vi "Nov_30.vi"() -> ()   [LabVIEW 2020]
uses:
  <vilib>/Utility/error.llb/DialogType.ctl
  <vilib>/Analysis/3filter.llb/Filter Passband Type.ctl
  <vilib>/DAQmx/read.llb/DAQmx Read (Analog 1D DBL NChan 1Samp).vi
  <vilib>/DAQmx/create/channels.llb/DAQmx Create Channel (AI-Voltage-Basic).vi
  <vilib>/DAQmx/configure/timing.llb/DAQmx Timing (Sample Clock).vi
  <vilib>/DAQmx/miscellaneous.llb/DAQmx Fill In Error Info.vi
  <vilib>/Analysis/3filter.llb/Butterworth Filter (DBL).vi
  <vilib>/Utility/file.llb/Write Delimited Spreadsheet (string).vi
  <vilib>/Utility/file.llb/Write Delimited Spreadsheet (DBL).vi
  <vilib>/Analysis/NI_AALBase.lvlib
panel:
  in  "Motor Enable":bool
  out "Swing (Consumer Loop)":bool
  in  "Motor Trottle":dbl(slide) scale=0.0..5.0
  in  "Master Stop":bool
  out "Consumer Loop Speed":u32
  out "Producer Loop Speed":u32
  out "Swing":bool
  out "Force Plate":dynamicdata(graph)
  out "Accelerometers":dynamicdata(graph)
  out "Enlapsed Time (sec)":dbl
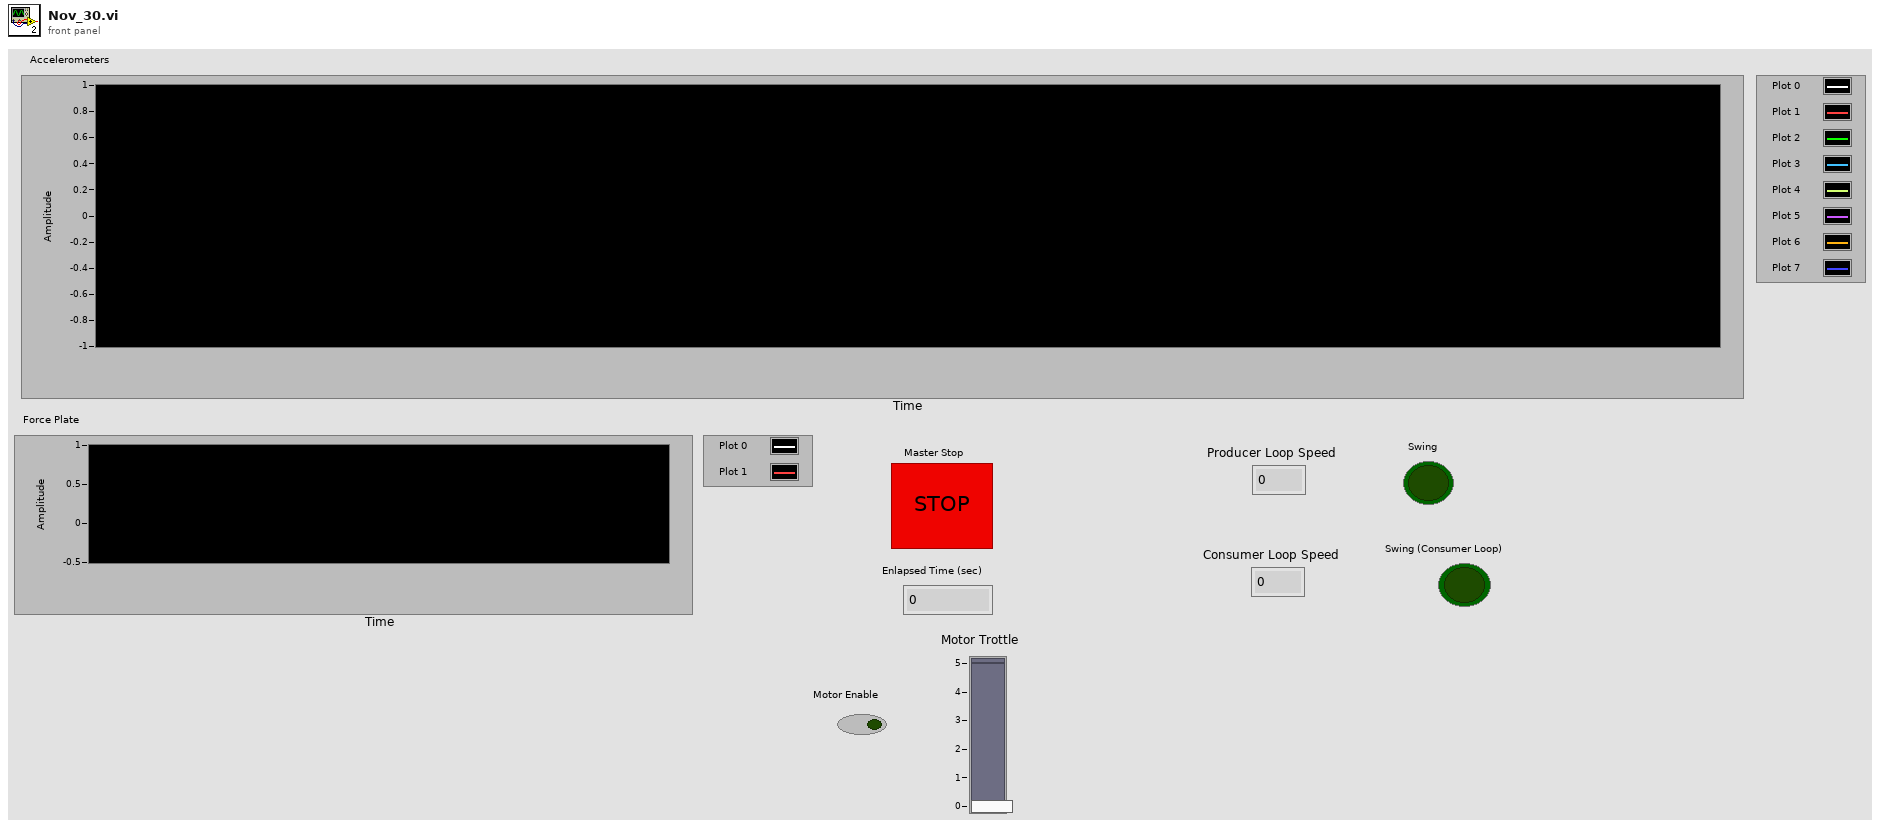
[diagram p1: front panel]
types:
  T1 = typedef "DialogType.ctl" = u16
  T2 = typedef "NI_AALBase.lvlib/Filter Passband Type.ctl" = enum32{"Lowpass", "Highpass", "Bandpass", "Bandstop"}
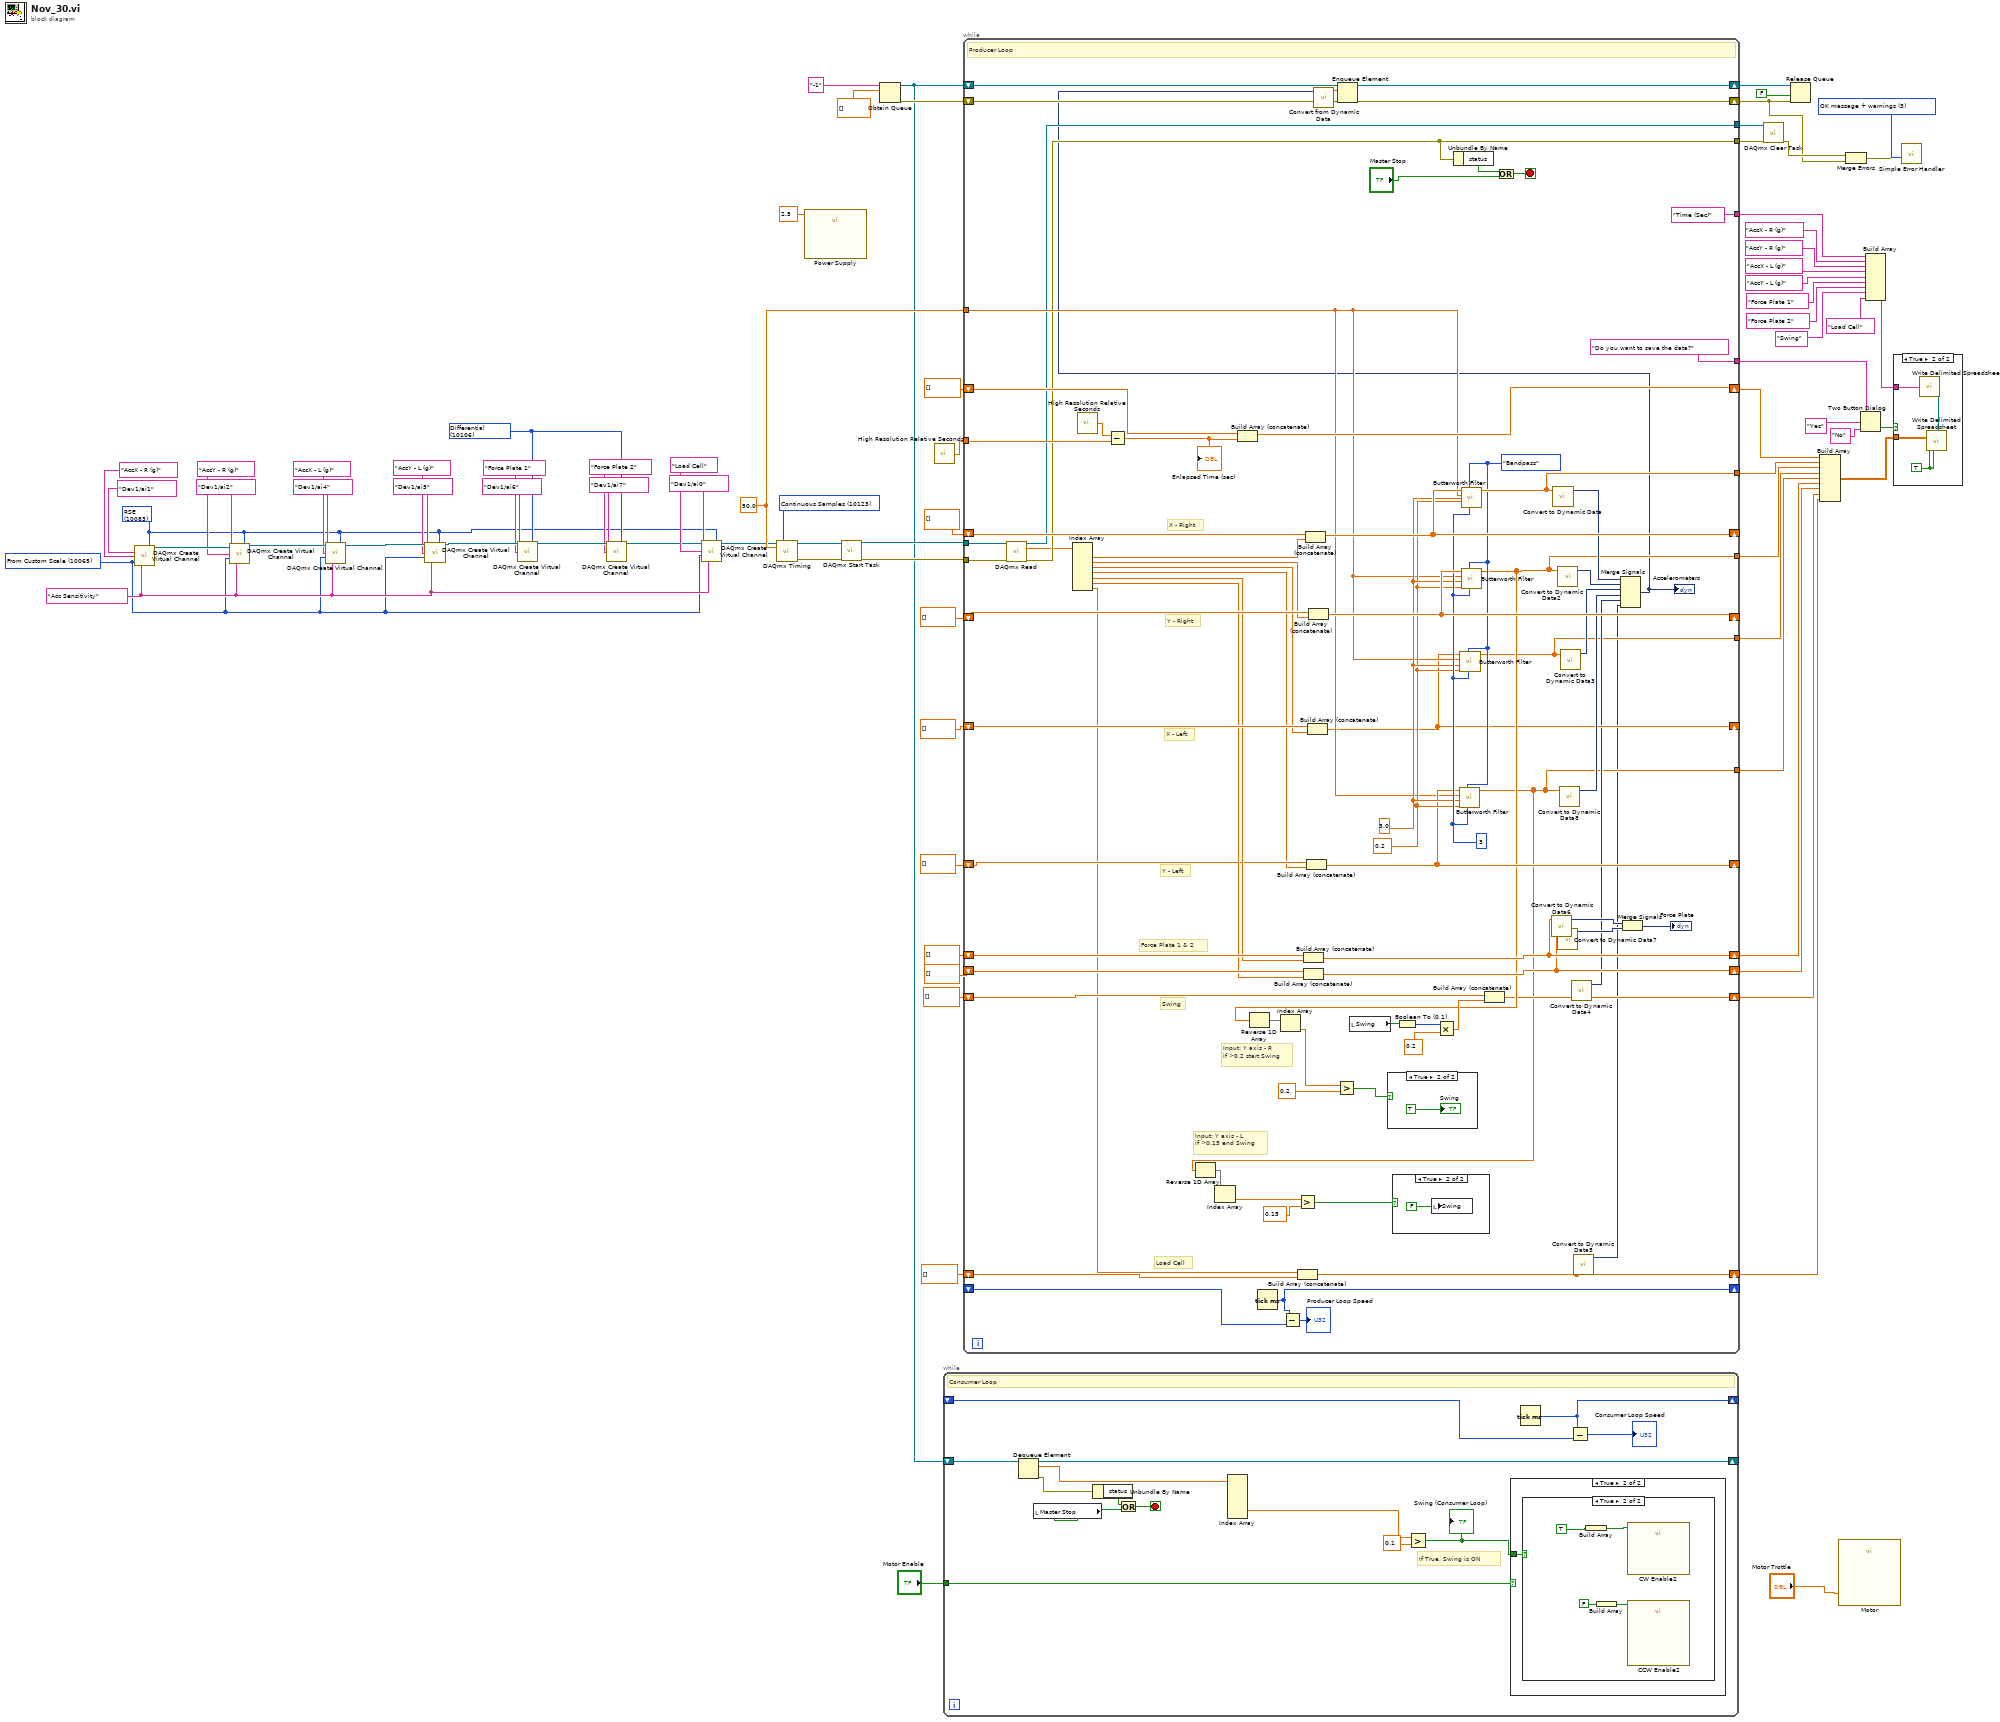
[diagram p0: block diagram]
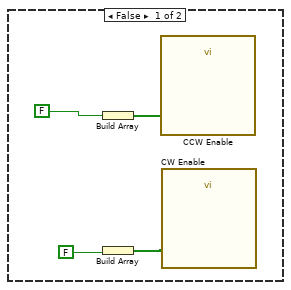
[diagram p3: hidden frame]
diagram:
  w17 = T1 3 items=["no dialog", "OK message", "continue or stop message", "OK message + warnings", "continue/stop + warnings"] ("type of dialog (OK msg:1)")
  w4 = 10065 items=["Volts"=10348, "From Custom Scale"=10065] ("units")
  w5 = tag "Acc Sensitivity" ("custom scale name")
  w27 = 10106 items=["Default"=-1, "RSE"=10083, "NRSE"=10078, "Differential"=10106, "Pseudodifferential"=12529] ("input terminal configuration")
  w49 = 10123 items=["Finite Samples"=10178, "Continuous Samples"=10123, "Hardware Timed Single Point"=12522] ("sample mode")
  w44 = 50.0 ("rate")
  w8 = 10083 items=["Default"=-1, "RSE"=10083, "NRSE"=10078, "Differential"=10106, "Pseudodifferential"=12529] ("input terminal configuration")
  n1 = call-poly <vilib>:"DAQmx Create Virtual Channel.vi"("input terminal configuration"=w8, "physical channels"=tag "Dev1/ai1" ("Physical channels"), "name to assign"="AccX - R (g)", "units"=w4, "custom scale name"=w5) -> ("task out"=w43:refnum<k21>)  [unwired: 9 in, 1 out]
  n2 = call-poly <vilib>:"DAQmx Create Virtual Channel.vi"("task in"=w43, "input terminal configuration"=w8, "physical channels"=tag "Dev1/ai2", "name to assign"="AccY - R (g)", "units"=w4, "custom scale name"=w5) -> ("task out"=w42:refnum<k21>)  [unwired: 8 in, 1 out]
  n3 = call-poly <vilib>:"DAQmx Create Virtual Channel.vi"("task in"=w42, "input terminal configuration"=w8, "physical channels"=tag "Dev1/ai4", "name to assign"="AccX - L (g)", "units"=w4, "custom scale name"=w5) -> ("task out"=w41:refnum<k21>)  [unwired: 8 in, 1 out]
  n4 = call-poly <vilib>:"DAQmx Create Virtual Channel.vi"("task in"=w41, "input terminal configuration"=w8, "physical channels"=tag "Dev1/ai5", "name to assign"="AccY - L (g)", "units"=w4, "custom scale name"=w5) -> ("task out"=w40:refnum<k21>)  [unwired: 8 in, 1 out]
  n5 = call-poly <vilib>:"DAQmx Create Virtual Channel.vi"("task in"=w40, "input terminal configuration"=w27, "physical channels"=tag "Dev1/ai6", "name to assign"="Force Plate 1" ("element")) -> ("task out"=w34:refnum<k21>)  [unwired: 10 in, 1 out]
  n6 = call-poly <vilib>:"DAQmx Create Virtual Channel.vi"("task in"=w34, "input terminal configuration"=w27, "physical channels"=tag "Dev1/ai7", "name to assign"="Force Plate 2" ("element")) -> ("task out"=w7:refnum<k21>)  [unwired: 10 in, 1 out]
  n7 = call-poly <vilib>:"DAQmx Create Virtual Channel.vi"("task in"=w7, "input terminal configuration"=w8, "physical channels"=tag "Dev1/ai0", "name to assign"="Load Cell", "units"=w4, "custom scale name"=w5) -> ("task out"=w6:refnum<k21>)  [unwired: 8 in, 1 out]
  n8 = call-poly <vilib>:"DAQmx Timing.vi"("task/channels in"=w6, "sample mode"=w49, "rate"=w44) -> ("task out"=w48:refnum<k21>, "error out"=w47:errorcluster)  [unwired: 11 in]
  n9 = call "Power Supply"("data"=2.5) -> ()  [unwired: 17 in, 2 out]
  n10 = call <vilib>:"DAQmx Start Task.vi"("task/channels in"=w48, "error in"=w47) -> ("task out"=w46:refnum<k21>, "error out"=w45:errorcluster)  [unwired: 12 in]
  n11 = Obtain Queue(name (unnamed)="-1", element data type=dbl[] []) -> (queue out=w13:refnum<queue>, error out=w22:errorcluster)  [unwired: 3 in, 1 out]
  n12 = call <vilib>:"High Resolution Relative Seconds.vi"() -> ("relative seconds"=w80:dbl)
  n13 = while {
    shift-right: [w93] -> _
    shift-left: w13 -> [w94]
    shift-right: [w90] -> _
    shift-left: _ -> [w91]
    tunnel: "Motor Enable" -> [w81]
    stop <- w88 stop-if-true
    # "If True, Swing is ON"
    # "Consumer Loop"
    n14 = Dequeue Element(queue=w94) -> (queue out=w93:refnum<queue>, element=w85:dbl[], error out=w87:errorcluster)  [unwired: 2 in, 1 out]
    n15 = local read "Master Stop"() -> (w86:bool)
    n16 = Unbundle By Name(w87) -> ("status"=w89:bool)
    n17 = Or(x=w89, y=w86) -> (x .or. y?=w88:bool)
    n18 = Index Array(array=w85) -> (element #5=w84:dbl)  [unwired: 6 in, 5 out]
    n19 = Greater?(x=w84, y=0.1) -> (0:w82:bool)
    "Swing (Consumer Loop)" <- w82
    n20 = case shown="True" w81 {
      tunnel: w82 -> [_ w95]
      frame False {
      }
      frame True {
        n21 = case shown="True" w95 {
          frame False {
            n22 = Build Array(FALSE) -> (w99:bool[])
            n23 = Build Array(FALSE) -> (w97:bool[])
            n24 = call "CCW Enable"("data"=w99) -> ()  [unwired: 17 in, 2 out]
            n25 = call "CW Enable"("data"=w97) -> ()  [unwired: 17 in, 2 out]
          }
          frame True {
            n26 = Build Array "Build Array"(TRUE) -> (w102:bool[])
            n27 = Build Array(FALSE) -> (w101:bool[])
            n28 = call "CW Enable2"("data"=w102) -> ()  [unwired: 17 in, 2 out]
            n29 = call "CCW Enable2"("data"=w101) -> ()  [unwired: 17 in, 2 out]
          }
        }
      }
    }
    n30 = Tick Count (ms)() -> (millisecond timer value=w90:u32)
    n31 = Subtract(x=w90, y=w91) -> (x-y=→"Consumer Loop Speed":u32)
  }
  n32 = while {
    tunnel: w46 -> [w180]
    tunnel: w45 -> [w179]
    tunnel: w80 -> [w177]
    shift-right: [w161] -> w77
    shift-left: dbl[] [] -> [w175]
    shift-right: [w165] -> _
    shift-left: dbl[] [] -> [w174]
    shift-right: [w164] -> _
    shift-left: dbl[] [] -> [w173]
    tunnel: ["Time (Sec)"] -> w52
    tunnel: ["Do you want to save the data?" ("message")] -> w69
    shift-right: [w125] -> w56
    shift-left: dbl[] [] -> [w170]
    shift-right: [w126] -> _
    shift-left: dbl[] [] -> [w162]
    shift-right: [w151] -> w54
    shift-left: dbl[] [] -> [w154]
    shift-right: [w149] -> w55
    shift-left: dbl[] [] -> [w153]
    tunnel: [w147] -> w59
    tunnel: [w129] -> w58
    tunnel: [w121] -> w57
    shift-right: [w140] -> _
    shift-left: dbl[] [] -> [w139]
    tunnel: [w120] -> w53
    tunnel: w44 -> [w137]
    shift-right: [w131] -> _
    shift-left: _ -> [w130]
    shift-right: [w114] -> w21
    shift-left: w13 -> [w115]
    shift-right: [w112] -> w14
    shift-left: w22 -> [w113]
    tunnel: [w119] -> w19
    tunnel: [w116] -> w18
    shift-right: [w105] -> w2
    shift-left: dbl[] [] -> [w107]
    stop <- w117 stop-if-true
    w144 = 3 ("order")
    w142 = 0.2 ("low cutoff freq: fl")
    w143 = 3.0 ("high cutoff freq: fh")
    w138 = Filter_Passband_Type."Bandpass" ("filter type")
    # "X - Right"
    # "Y - Right"
    # "X - Left"
    # "Y - Left"
    # "Force Plate 1 & 2"
    # "Swing"
    # "Load Cell"
    # "Input: Y axis - L\nif >0.15 end Swing"
    # "Input: Y axis - R\nif >0.2 start Swing"
    # "Producer Loop"
    n33 = call-poly <vilib>:"DAQmx Read.vi"("task/channels in"=w180, "error in"=w179) -> ("task out"=w119:refnum<k21>, "data"=w111:dbl[], "error out"=w116:errorcluster)  [unwired: 11 in]
    n34 = Index Array(array=w111) -> (element #1=w136:dbl, element #2=w135:dbl, element #3=w134:dbl, element #4=w133:dbl, element #5=w145:dbl, element #6=w146:dbl, element #7=w106:dbl)  [unwired: 7 in]
    n35 = call <vilib>:"High Resolution Relative Seconds.vi"() -> ("relative seconds"=w178:dbl)
    n36 = Subtract(x=w178, y=w177) -> (x-y=w176:dbl)
    "Enlapsed Time (sec)" <- w176
    n37 = Build Array (concatenate)(w175, w176) -> (w161:dbl[])
    n38 = Tick Count (ms)() -> (millisecond timer value=w131:u32)
    n39 = Subtract(x=w131, y=w130) -> (x-y=→"Producer Loop Speed":u32)
    n40 = Build Array (concatenate)(w106, w107) -> (w105:dbl[])
    n41 = Build Array (concatenate)(w154, w145) -> (w151:dbl[])
    n42 = Build Array (concatenate)(w153, w146) -> (w149:dbl[])
    n43 = Build Array (concatenate)(w174, w136) -> (w165:dbl[])
    n44 = Build Array (concatenate)(w139, w133) -> (w140:dbl[])
    n45 = Build Array (concatenate)(w162, w134) -> (w126:dbl[])
    n46 = Build Array (concatenate)(w173, w135) -> (w164:dbl[])
    n47 = local read "Swing"() -> (w163:bool)
    n48 = Boolean To (0,1)(Boolean=w163) -> (0, 1=w168:i16)
    n49 = Multiply(x=w168, y=0.2) -> (x*y=w169:dbl)
    n50 = Unbundle By Name(w116) -> ("status"=w118:bool)
    n51 = call-poly <vilib>:"Butterworth Filter.vi"("order"=w144, "filter type"=w138, "low cutoff freq: fl"=w142, "high cutoff freq: fh"=w143, "sampling freq: fs"=w137, "X"=w140) -> ("Filtered X"=w120:dbl[])  [unwired: 2 in, 1 out]
    n52 = Reverse 1D Array(array=w120) -> (reversed array=w156:dbl[])
    n53 = Index Array(array=w156) -> (element=w155:dbl)  [unwired: 1 in]
    n54 = Greater?(x=w155, y=0.15) -> (0:w123:bool)
    n55 = case shown="True" w123 {
      frame False {
      }
      frame True {
        n56 = local write "Swing"(FALSE) -> ()
      }
    }
    n57 = call-poly <vilib>:"Butterworth Filter.vi"("order"=w144, "filter type"=w138, "low cutoff freq: fl"=w142, "high cutoff freq: fh"=w143, "sampling freq: fs"=w137, "X"=w126) -> ("Filtered X"=w121:dbl[])  [unwired: 2 in, 1 out]
    n58 = call-poly <vilib>:"Butterworth Filter.vi"("order"=w144, "filter type"=w138, "low cutoff freq: fl"=w142, "high cutoff freq: fh"=w143, "sampling freq: fs"=w137, "X"=w165) -> ("Filtered X"=w147:dbl[])  [unwired: 2 in, 1 out]
    n59 = call-poly <vilib>:"Butterworth Filter.vi"("order"=w144, "filter type"=w138, "low cutoff freq: fl"=w142, "high cutoff freq: fh"=w143, "sampling freq: fs"=w137, "X"=w164) -> ("Filtered X"=w129:dbl[])  [unwired: 2 in, 1 out]
    n60 = Reverse 1D Array(array=w129) -> (reversed array=w166:dbl[])
    n61 = Index Array(array=w166) -> (element=w128:dbl)  [unwired: 1 in]
    n62 = Greater?(x=w128, y=0.2) -> (0:w122:bool)
    n63 = case shown="True" w122 {
      frame False {
      }
      frame True {
        "Swing" <- TRUE
      }
    }
    n64 = Build Array (concatenate)(w170, w169) -> (w125:dbl[])
    n65 = Or(x=w118, y="Master Stop") -> (x .or. y?=w117:bool)
    n66 = call "Convert to Dynamic Data6"("Array"=w151) -> ("Dynamic Data Type"=w150:dynamicdata)  [unwired: 3 in]
    n67 = call "Convert to Dynamic Data"("Array"=w147) -> ("Dynamic Data Type"=w160:dynamicdata)  [unwired: 3 in]
    n68 = call "Convert to Dynamic Data2"("Array"=w129) -> ("Dynamic Data Type"=w159:dynamicdata)  [unwired: 3 in]
    n69 = call "Convert to Dynamic Data7"("Array"=w149) -> ("Dynamic Data Type"=w148:dynamicdata)  [unwired: 3 in]
    n70 = call "Convert to Dynamic Data8"("Array"=w120) -> ("Dynamic Data Type"=w141:dynamicdata)  [unwired: 3 in]
    n71 = call "Convert to Dynamic Data3"("Array"=w121) -> ("Dynamic Data Type"=w158:dynamicdata)  [unwired: 3 in]
    n72 = call "Convert to Dynamic Data4"("Array"=w125) -> ("Dynamic Data Type"=w124:dynamicdata)  [unwired: 3 in]
    n73 = call "Convert to Dynamic Data5"("Array"=w105) -> ("Dynamic Data Type"=w104:dynamicdata)  [unwired: 3 in]
    n74 = Merge Signals(w160, w159, w158, w141, w124, w104) -> (w109:dynamicdata)
    "Accelerometers" <- w109
    n75 = call "Convert from Dynamic Data"("Dynamic Data Type"=w109) -> ("Array"=w108:dbl[])  [unwired: 3 in]
    n76 = Enqueue Element(queue=w115, element=w108, error in (no error)=w113) -> (queue out=w114:refnum<queue>, error out=w112:errorcluster)  [unwired: 1 in, 1 out]
    n77 = Merge Signals(w150, w148) -> (→"Force Plate":dynamicdata)
  }
  n78 = call <vilib>:"DAQmx Clear Task.vi"("task in"=w19, "error in"=w18) -> ("error out"=w15:errorcluster)  [unwired: 13 out]
  n79 = Release Queue(queue=w21, force destroy? (F)=FALSE, error in (no error)=w14) -> ()  [unwired: 3 out]
  n80 = Build Array(w77, w59, w58, w57, w53, w54, w55, w56, w2) -> (w76:dbl[][])
  n81 = call "Motor"("data"="Motor Trottle") -> ()  [unwired: 17 in, 2 out]
  n82 = Merge Errors(w15, w14) -> (w16:errorcluster)
  n83 = Two Button Dialog(message=w69, 1:"No" ("F button name (\"Cancel\")"), 2:"Yes" ("T button name (\"OK\")")) -> (T button?=w72:bool)
  n84 = Build Array(w52, "AccX - R (g)", "AccY - R (g)", "AccX - L (g)", "AccY - L (g)", "Force Plate 1" ("element"), "Force Plate 2" ("element"), "Swing" ("element"), "Load Cell" ("element")) -> (w75:string[])
  n85 = case shown="True" w72 {
    tunnel: w76 -> [_ w186]
    tunnel: w75 -> [_ w185]
    frame False {
    }
    frame True {
      w184 = TRUE ("transpose? (no:F)")
      n86 = call-poly <vilib>:"Write Delimited Spreadsheet.vi"("1D data"=w185) -> ("new file path (Not A Path if cancelled)"=w183:path)  [unwired: 13 in, 1 out]
      n87 = call-poly <vilib>:"Write Delimited Spreadsheet.vi"("file path (dialog if empty)"=w183, "2D data"=w186, "append to file? (new file:F)"=w184, "transpose? (no:F)"=w184) -> ()  [unwired: 10 in, 2 out]
    }
  }
  n88 = call <vilib>:"Simple Error Handler.vi"("type of dialog (OK msg:1)"=w17, "error in (no error)"=w16) -> ()  [unwired: 8 out]
